vi "启动界面.vi"() -> ()   [LabVIEW 2015]
doc: "This example uses VI Server to display a splash screen for your main application while all its subVIs load into memory. This is useful if you have a large application that takes a while to load, because the splash screen can display your company information, along with an indicator displaying the load status.\n\nThe VI uses a hidden string indicator in conjuction with a horizontal bar control to achieve the desired user interface."
panel:
  out "Current Status":string
  out "String":string
  out "Slide":u8(slide) scale=0.0..5.0
  # "启动界面..."
  # "直流伺服电机位置控制系统框图"
  # "给定值"
  # "位移"
  # "PID控制算法"
  # "D/A"
  # "减速器"
  # "伺服电源"
  # "直流伺服电机"
  # "滚珠丝杆"
  # "负载"
  # "位移传感器"
  # "A/D"
  # "直流电机位置控制系统"
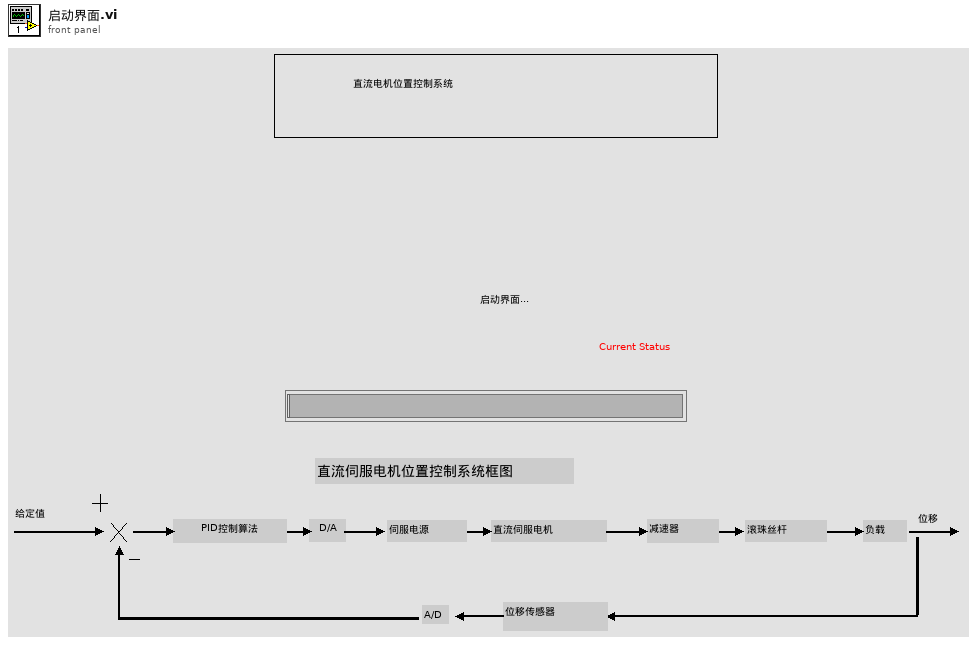
[diagram p1: front panel]
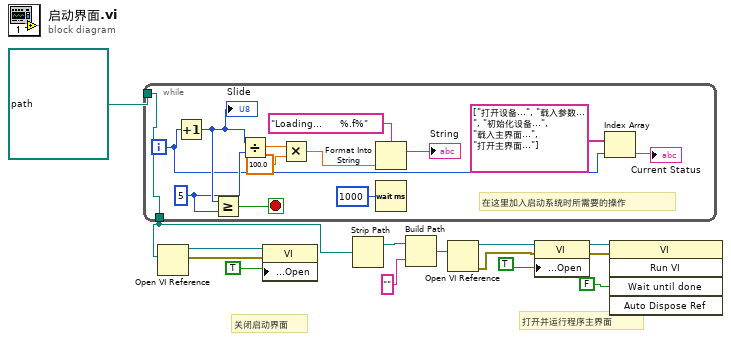
[diagram p0: block diagram]
diagram:
  # "打开并运行程序主界面"
  # "关闭启动界面"
  n1 = while {
    tunnel: path "C:/Documents and Settings/Heego/桌面/源程序/总程序.vi" -> [w20]
    tunnel: [w20] -> w2
    i -> [w16]
    stop <- w25 stop-if-true
    w22 = 5 ("y")
    # "在这里加入启动系统时所需要的操作"
    n2 = Increment(x=w16) -> (x+1=w24:i32)
    "Slide" <- w24
    n3 = Greater Or Equal?(x=w24, y=w22) -> (x >= y?=w25:bool)
    n4 = Divide(x=w24, y=w22) -> (x/y=w23:dbl)
    n5 = Multiply(x=w23, y=100.0) -> (x*y=w19:dbl)
    n6 = Format Into String(format string="Loading...      %.f%", w19) -> (resulting string=→"String":string)  [unwired: 2 in, 1 out]
    n7 = Wait (ms)(milliseconds to wait=u32 1000) -> ()  [unwired: 1 out]
    n8 = Index Array(array=string[] ["打开设备...", "载入参数...", "初始化设备...", "载入主界面...", "打开主界面..."], index=w16) -> (element=→"Current Status":string)
  }
  n9 = Open VI Reference(vi path=w2) -> (vi reference=w13:refnum<vi>, error out=w11:errorcluster)  [unwired: 5 in]
  n10 = property on="Property Node" class="VI"(reference=w13, error in=w11, "Front Panel Window:Open"=TRUE) -> ()  [unwired: 2 out]
  n11 = Strip Path(path=w2) -> (stripped path=w3:path)  [unwired: 1 out]
  n12 = Build Path(base path=w3, name or relative path="") -> (appended path=w4:path)
  n13 = Open VI Reference(vi path=w4) -> (vi reference=w5:refnum<vi>, error out=w6:errorcluster)  [unwired: 5 in]
  n14 = property on="Property Node" class="VI"(reference=w5, error in=w6, "Front Panel Window:Open"=TRUE) -> (reference out=w8:refnum<vi>, error out=w9:errorcluster)
  n15 = invoke class="VI" method="Run VI"(reference=w8, error in=w9, "Wait until done"=FALSE) -> ()  [unwired: 2 in, 5 out]
